vi "Probe-U32-Bool.vi"(9 "Set-Val":bool, 10 "Bool-Val":bool, 11 "U32-Val":u32) -> (2 "Probe-Bool":bool[](array[boolean]), 3 "Probe-U32":u32[](array[numeric]))   [LabVIEW 2014]
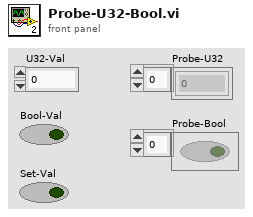
[diagram p1: front panel]
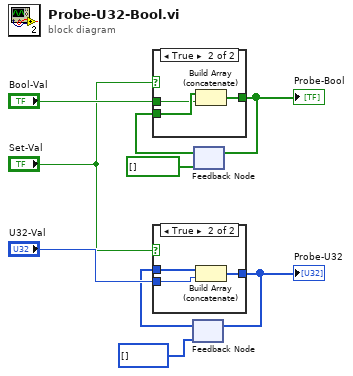
[diagram p0: block diagram]
diagram:
  n1 = feedback #1(i32[] []) -> (w1:u32[])
  n2 = case shown="True" "Set-Val" {
    tunnel: w1 -> [w10 w13]
    tunnel: "U32-Val" -> [_ w12]
    tunnel: [w10 w11] -> w5
    frame False {
    }
    frame True {
      n3 = Build Array (concatenate)(w13, w12) -> (w11:u32[])
    }
  }
  "Probe-U32" <- w5
  n4 = feedback-in #1(w5) -> ()
  n5 = feedback #2(bool[] []) -> (w3:bool[])
  n6 = case shown="True" "Set-Val" {
    tunnel: w3 -> [w14 w17]
    tunnel: "Bool-Val" -> [_ w16]
    tunnel: [w14 w15] -> w6
    frame False {
    }
    frame True {
      n7 = Build Array (concatenate)(w17, w16) -> (w15:bool[])
    }
  }
  "Probe-Bool" <- w6
  n8 = feedback-in #2(w6) -> ()
